vi "beginPassToStrikerPlay.vi"(8 "error in (no error)":errorcluster, 10 "Game":refnum<class "Game.lvclass">, 11 "PassToStriker in":refnum<class "PassToStriker.lvclass">) -> (0 "error out":errorcluster, 2 "BeginPassToStriker?":bool, 3 "PassToStriker out":refnum<class "PassToStriker.lvclass">)   [LabVIEW 2023, in "PassToStriker.lvclass"]
uses:
  PassToStriker.lvclass
  Game_class/Game.lvclass
  Utilities_class/Utilities.lvclass
  Referee_class/command_interpreted.ctl
  Team_class/OffensivePlay.ctl
  Game_class/Game.lvclass/Game.ctl
  Team_class/Team.lvclass/Team.ctl
  Referee_class/Referee.lvclass/Referee.ctl
  Game_class/Read Referee.vi
  Referee_class/Read command_interpreted.vi
  Game_class/Read OffensiveTeam.vi
  Team_class/Read RobotRef.vi
  Team_class/Read OffensivePlay.vi
  Ally_class/Ally.lvclass
  C:/Users/roboi/Downloads/VSS_AI-Larc2023/Team_class/Team.lvclass
  Robot_class/Robot.lvclass
  Referee_class/Referee.lvclass
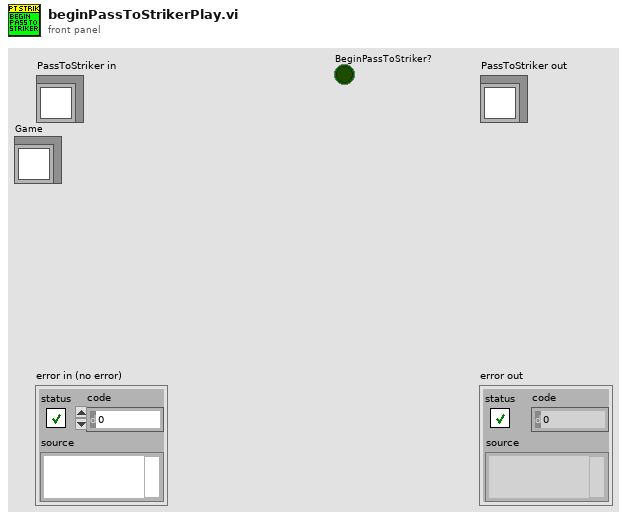
[diagram p1: front panel]
types:
  T1 = typedef "OffensivePlay.ctl" = enum16{"TableWithStriker", "TableWith2ndStrikerPlay", "PrepareDoublePass", "PrepareRollToPass", "SimplePass", "PreparePass", "PassToStriker", "BallOutOfField", "PassTo2ndStriker", "StopOffensive", "Prepare Penalty Enemy", "EnemyPossessionAtEnemyField", "EnemyPossesionAtOurField", "TestPlay", "PreparePenaltyAlly", "KickPenaltyAlly", "PrepareKickoffAlly", "PrepareKickoffEnemy", "IndirectEnemy", "DirectEnemy", "NormalGame", "DirectKick", "Pass", "Halt", "Timeout", "PassPlay", "PenaltyEnemy"}
  T2 = typedef "command_interpreted.ctl" = enum16{"Goal Ally", "Goal Enemy", "Ball Placement Enemy", "Ball Placement Ally", "Normal Half Time", "Extra Time  Break", "Extra Half Time", "None", "Post Game", "PKA Normal Start", "Prepare Kickoff Ally", "PKE Normal Start", "Prepare Kickoff Enemy", "Force Start", "Halt", "Timeout", "Prepare Penalty Ally", "Prepare Penalty Enemy", "PPA NormalStart", "PPE Normal Start", "Indirect Free Ally", "Direct Free Enemy", "Direct Free Ally", "Indirect Free Enemy", "Stop"}
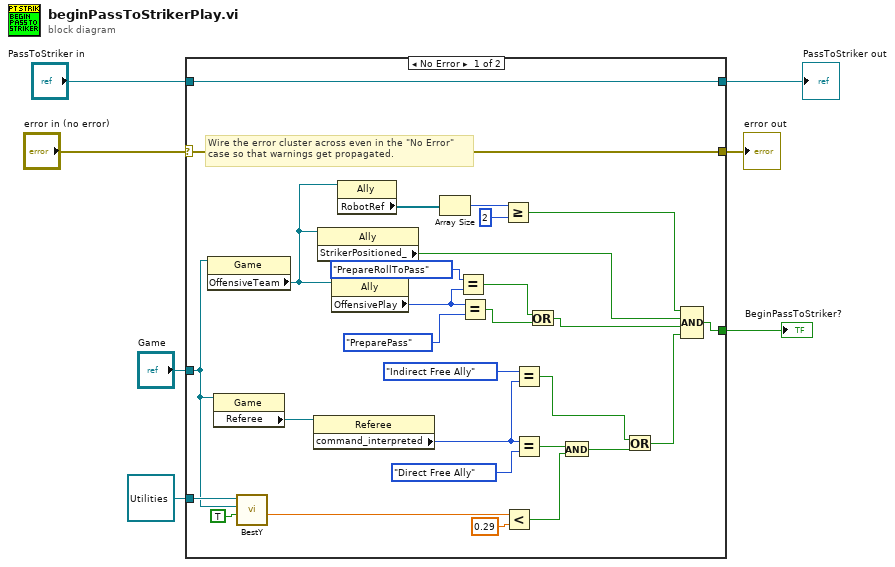
[diagram p0: block diagram]
diagram:
  n1 = case shown="No Error" "error in (no error)" {
    selector: "error in (no error)" -> [w35 w38]
    tunnel: [w35 w38] -> w6
    tunnel: [w36 w37] -> w4
    tunnel: "PassToStriker in" -> [w36 w37]
    tunnel: "Game" -> [w25 _]
    tunnel: refnum<class "Utilities.lvclass"> refnum ("Utilities.lvclass") -> [w26 _]
    tunnel: [w24 _] -> w1
    frame No Error {
      # "Wire the error cluster across even in the \"No Error\"\ncase so that warnings get propagated."
      n2 = property class="Game"(reference=w25) -> ("OffensiveTeam"=w13:refnum<class "Ally.lvclass">)  [unwired: 1 in, 2 out]
      n3 = property class="Game"(reference=w25) -> ("Referee"=w34:refnum<class "Referee.lvclass">)  [unwired: 1 in, 2 out]
      n4 = call "BestY.vi"("Utilities in"=w26, "Game"=w25, "inimigos"=TRUE) -> ("Gap kick"=w28:dbl)  [unwired: 2 in, 4 out]
      n5 = property class="Referee"(reference=w34) -> ("command_interpreted"=w32:T2)  [unwired: 1 in, 2 out]
      n6 = property class="Ally"(reference=w13) -> ("StrikerPositioned_"=w23:bool)  [unwired: 1 in, 2 out]
      n7 = property class="Ally"(reference=w13) -> ("OffensivePlay"=w18:T1)  [unwired: 1 in, 2 out]
      n8 = property class="Ally"(reference=w13) -> ("RobotRef"=w12:refnum<class "Robot.lvclass">[])  [unwired: 1 in, 2 out]
      n9 = Array Size(array=w12) -> (size(s)=w11:i32)
      n10 = Equal?(x=OffensivePlay."PrepareRollToPass" ("OffensivePlay"), y=w18) -> (x = y?=w15:bool)
      n11 = Equal?(x=w18, y=OffensivePlay."PreparePass" ("OffensivePlay")) -> (x = y?=w16:bool)
      n12 = Greater Or Equal?(x=w11, y=2) -> (x >= y?=w9:bool)
      n13 = Less?(x=w28, y=0.29 ("Gap kick")) -> (x < y?=w27:bool)
      n14 = Equal?(x=command_interpreted."Indirect Free Ally" ("command_interpreted"), y=w32) -> (x = y?=w20:bool)
      n15 = Equal?(x=w32, y=command_interpreted."Direct Free Ally" ("command_interpreted")) -> (x = y?=w22:bool)
      n16 = Or(x=w15, y=w16) -> (x .or. y?=w14:bool)
      n17 = And(x=w22, y=w27) -> (x .and. y?=w21:bool)
      n18 = Or(x=w20, y=w21) -> (x .or. y?=w8:bool)
      n19 = Compound Arithmetic op=AND(w9, w23, w14, w8) -> (w24:bool)
    }
    frame Error {
    }
  }
  "error out" <- w6
  "PassToStriker out" <- w4
  "BeginPassToStriker?" <- w1
